vi "Get new SerNumber from XLS(HasHeader）.vi"(11 "file path (dialog if empty)":path caption="文件路径 （空时为对话框）") -> (3 "SerNumber":i32)   [LabVIEW 2018]
doc: "从本地xls文件中获取最新流水号；\n若本地文件无表头，则须在最新流水后＋1；"
uses:
  <vilib>/Utility/file.llb/Read Delimited Spreadsheet (string).vi
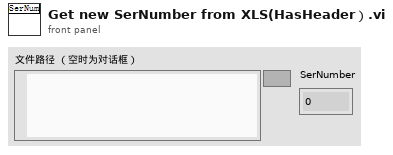
[diagram p1: front panel]
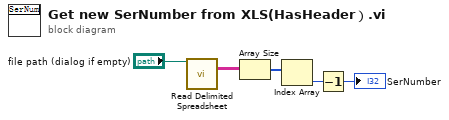
[diagram p0: block diagram]
diagram:
  n1 = call-poly <vilib>:"Read Delimited Spreadsheet.vi"("file path (dialog if empty)"="file path (dialog if empty)") -> ("all rows"=w3:string[][])  [unwired: 9 in, 5 out]
  n2 = Array Size(array=w3) -> (size(s)=w5:i32[])
  n3 = Index Array(array=w5) -> (element=w2:i32)  [unwired: 1 in]
  n4 = Decrement(x=w2) -> (x-1=→"SerNumber":i32)
